vi "Copy Value.vi"(10 "From":refnum<class "Type.lvclass">, 11 "String in":refnum<class "String.lvclass">) -> (2 "error out":errorcluster, 3 "String out":refnum<class "String.lvclass">)   [LabVIEW 2020, in "Conditu2.lvlib" / "Columns.lvlib" / "String.lvclass"]
uses:
  String.lvclass
  C:/dev/lv20CE/lv-conditum-tools/Conditum-Clone/Columns/Type/Type.lvclass
  Type/Type.lvclass
  String.lvclass/String.ctl
  Type/Type.lvclass/Type.ctl
  Type/Clear NULL.vi
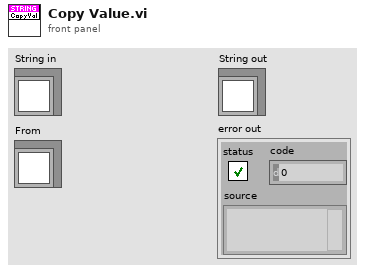
[diagram p1: front panel]
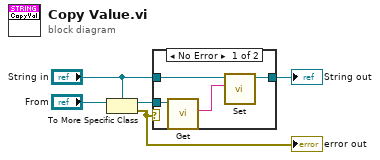
[diagram p0: block diagram]
diagram:
  n1 = To More Specific Class(target class="String in", reference="From") -> (specific class reference=w5:refnum<class "String.lvclass">, error out=w3:errorcluster)  [unwired: 1 in]
  "error out" <- w3
  n2 = case shown="No Error" w3 {
    tunnel: w5 -> [w9 _]
    tunnel: "String in" -> [w7 w10]
    tunnel: [w6 w10] -> w4
    frame No Error {
      n3 = call "Get.vi"("String in"=w9) -> ("Value"=w8:string)  [unwired: 10 in]
      n4 = call "Set.vi"("Value"=w8, "String in"=w7) -> ("String out"=w6:refnum<class "String.lvclass">)  [unwired: 9 in]
    }
    frame Error {
    }
  }
  "String out" <- w4
